vi "KE_Reverse.vi"(8 "error in (no error)":errorcluster, 11 "Instruments in":refnum<class "Instruments.lvclass">) -> (0 "error out":errorcluster, 2 "Current":dbl, 3 "Instruments out":refnum<class "Instruments.lvclass">)   [LabVIEW 2012, in "Instruments.lvclass"]
uses:
  Instruments.lvclass
  Instruments.lvclass/Instruments.ctl
  Instruments/Drivers/ke236/KE236.LLB/Keith 236 Operate/Standby.vi
panel:
  out "device dependent errors":string
  in  "integration time (medium:1)":u16(ring)=1 items=["fast perod", "medium period", "line cycle period @ 50Hz", "line cycle period @ 60Hz"]
  out "?":T1(array[cluster])
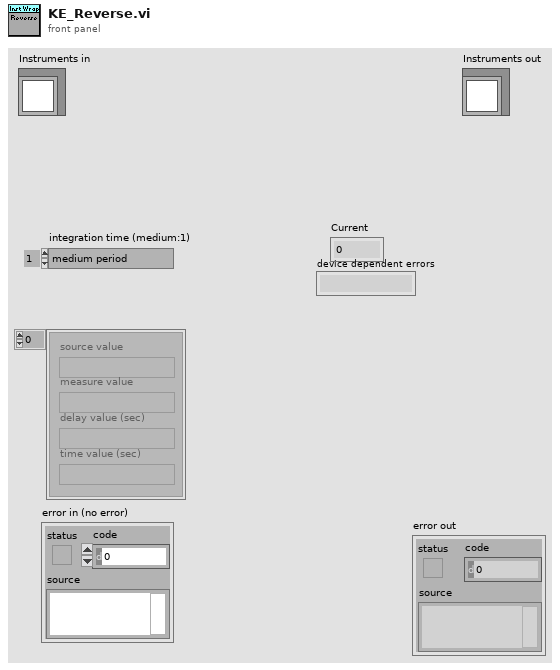
[diagram p1: front panel]
types:
  T1 = cluster{"source value":string, "measure value":string, "delay value (sec)":string, "time value (sec)":string}[]
  T2 = typedef "SMUParam.ctl" = cluster{"Start Current,mA":dbl, "Stop Current,mA":dbl, "Voltage Compliance,V":dbl, "GPIB":string, "VISA resource name":refnum<visa-resource-name>}
  T3 = cluster{"error":bool, "code":i32, "source":string}
  T4 = cluster{"source value":string, "measure value":string, "delay value (sec)":string, "time value (sec)":string}
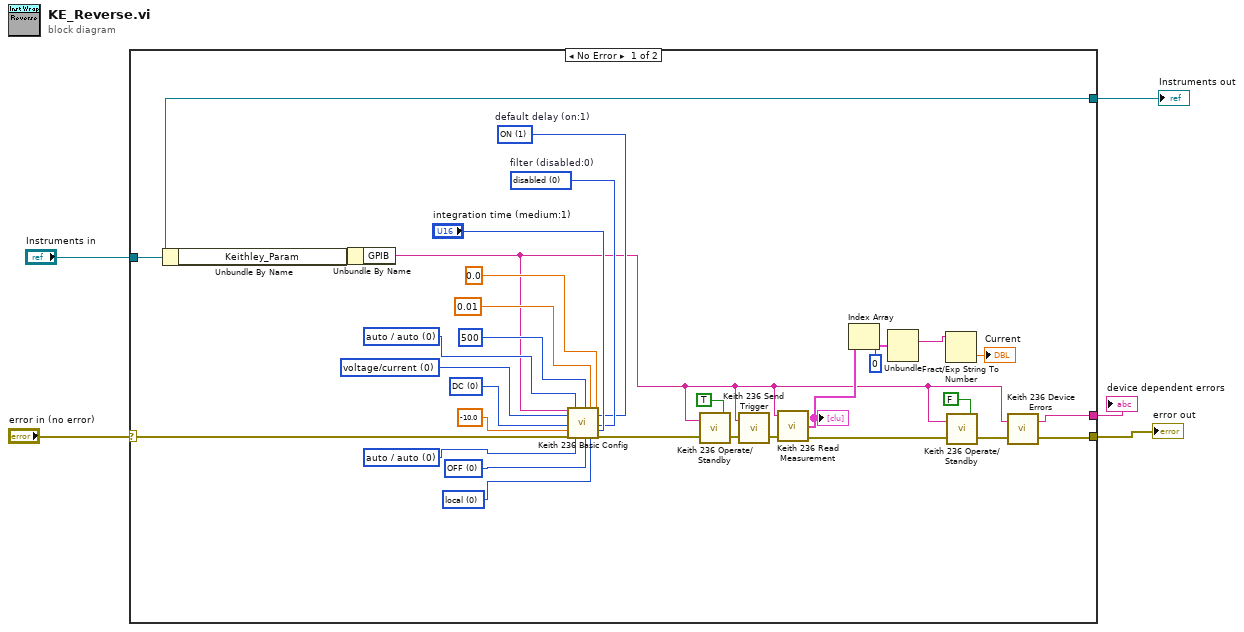
[diagram p0: block diagram]
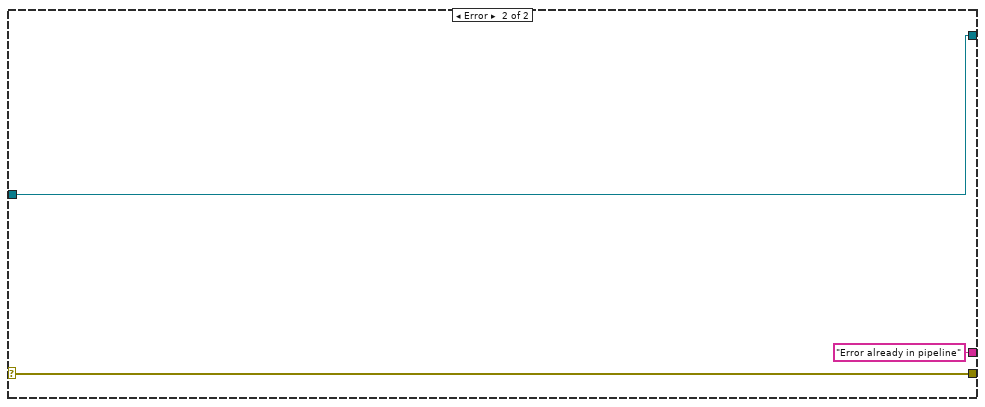
[diagram p2: hidden frame]
diagram:
  n1 = case shown="No Error" "error in (no error)" {
    selector: "error in (no error)" -> [w24 w39]
    tunnel: [w7 w39] -> w4
    tunnel: [w22 w38] -> w2
    tunnel: "Instruments in" -> [w22 w38]
    tunnel: [w6 "Error already in pipeline" ("device dependent errors")] -> w1
    frame No Error {
      w26 = u16 1 items=["OFF", "ON"]  # default delay (on:1)
      w27 = u16 0 items=["disabled", "2 readings", "4 readings", "8 readings", "16 readings", "32 readings"]  # filter (disabled:0)
      w30 = u16 0 items=["local", "remote"] ("sense (local:0)")
      w31 = u16 0 items=["OFF", "ON"] ("suppression (off:0)")
      w32 = u16 0 items=["auto / auto", "1 nA / 1.1 V", "10 nA / 11 V", "100 nA / 110 V", "0.001 mA / 110 V", "0.01 mA / 110 V", "0.1 mA / 110 V", "1 mA / 110 V", "10 mA / 110 V", "100 mA / 110 V"] ("compliance/\nmeasurement range (auto:0)")
      w33 = u16 0 items=["DC", "sweep"] ("function (DC:0)")
      w34 = u16 0 items=["voltage/current", "current/voltage"] ("source/measure (V/I:0)")
      w35 = u16 0 items=["auto / auto", "1 nA / 1.1 V", "10 nA / 11 V", "100 nA / 110 V", "0.001 mA / 110 V", "0.01 mA / 110 V", "0.1 mA / 110 V", "1 mA / 110 V", "10 mA / 110 V", "100 mA / 110 V"] ("source range\nI source / V source (auto:0)")
      n2 = Unbundle By Name(w22) -> ("Keithley_Param"=w36:T2)
      n3 = Unbundle By Name(w36) -> ("GPIB"=w8:string)
      n4 = call "Keith 236 Basic Config.vi"("GPIB address"=w8, "source/measure (V/I:0)"=w34, "function (DC:0)"=w33, "source level"=-10.0, "error in"=w24, "source range\nI source / V source (auto:0)"=w35, "compliance/\nmeasurement range (auto:0)"=w32, "timeout ms"=u32 500, "suppression (off:0)"=w31, "current \ncompliance level"=0.01 ("current \ncompliance level"), "sense (local:0)"=w30, "DC delay (sec)"=0.0, "default delay (on:1)"=w26, "filter (disabled:0)"=w27, "integration time (medium:1)"="integration time (medium:1)") -> ("error out"=w13:T3)  [unwired: 4 in]
      n5 = call "Keith 236 Operate/Standby.vi"("source"=TRUE, "error in"=w13, "GPIB address"=w8) -> ("error out"=w19:T3)
      n6 = call "Keith 236 Send Trigger.vi"("GPIB address"=w8, "error in"=w19) -> ("error out"=w20:T3)
      n7 = call "Keith 236 Read Measurement.vi"("error in"=w20, "GPIB address"=w8) -> ("error out"=w10:T3, "display"=w18:T1)  [unwired: 2 out]
      "?" <- w18
      n8 = Index Array(array=w18, index=0) -> (element=w16:T4)
      n9 = Unbundle(w16) -> ("measure value"=w15:string)  [unwired: 3 out]
      n10 = Fract/Exp String To Number(string=w15) -> (number=→"Current":dbl)  [unwired: 3 in, 1 out]
      n11 = call "Keith 236 Operate/Standby.vi"("source"=FALSE, "error in"=w10, "GPIB address"=w8) -> ("error out"=w9:T3)
      n12 = call "Keith 236 Device Errors.vi"("error in"=w9, "GPIB address"=w8) -> ("error out"=w7:T3, "device dependent errors"=w6:string)
    }
    frame Error {
    }
  }
  "error out" <- w4
  "Instruments out" <- w2
  "device dependent errors" <- w1
